vi "ListMenuActivation.vi"(0 "ListBox in":refnum<vi>, 1 "MenuRef":refnum<k9>, 2 "Point":T1) -> (14 "Menu Items":string[](array[string]), 19 "Discard Event?":bool)   [LabVIEW 2014, in "XListGraph.lvlib" / "XListGraph.xctl"]
uses:
  XListGraph.xctl
  <vilib>/Utility/miscctls.llb/LVPositionTypeDef.ctl
  <userlib>/_OpenG.lib/array/array.llb/Index 1D Array Elements (String)__ogtk.vi
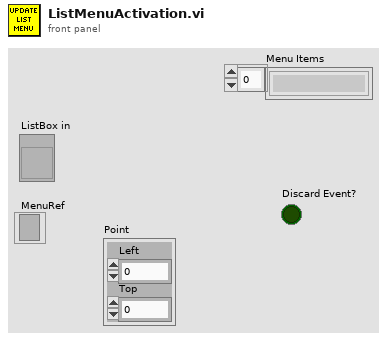
[diagram p1: front panel]
types:
  T1 = typedef "LVPositionTypeDef.ctl" = cluster{"Left":i32, "Top":i32}
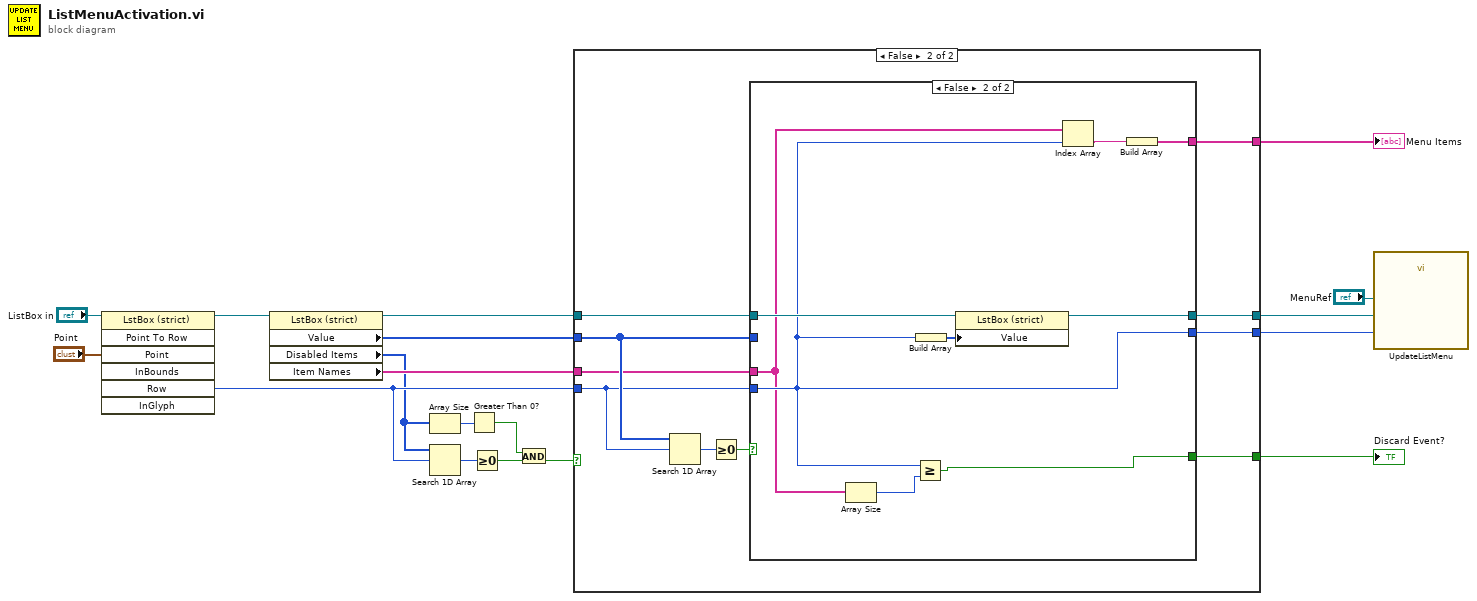
[diagram p0: block diagram]
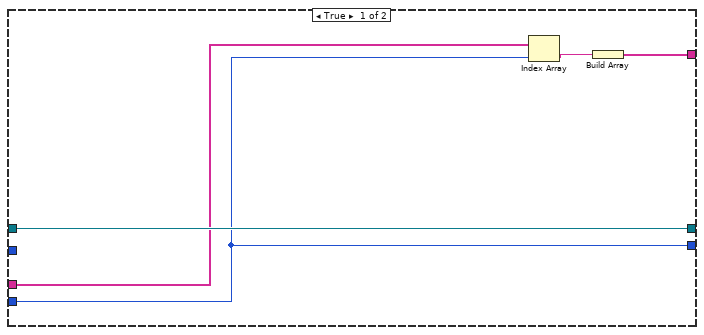
[diagram p2: hidden frame]
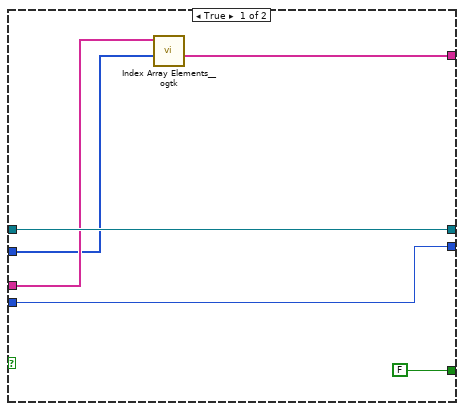
[diagram p3: hidden frame]
diagram:
  n1 = invoke on="Invoke Node" class="LstBox (strict)" method="Point To Row"(reference="ListBox in", "Point"="Point") -> (reference out=w15:refnum<vi>, "Row"=w11:i32)  [unwired: 5 in, 5 out]
  n2 = property class="LstBox (strict)"(reference=w15) -> (reference out=w14:refnum<vi>, "Value"=w18:i32[], "Disabled Items"=w4:i32[], "Item Names"=w16:string[])  [unwired: 1 in, 1 out]
  n3 = Array Size(array=w4) -> (size(s)=w2:i32)
  n4 = Search 1D Array(1D array=w4, element=w11) -> (index of element=w10:i32)  [unwired: 1 in]
  n5 = Greater Than 0?(x=w2) -> (x > 0?=w1:bool)
  n6 = Greater Or Equal To 0?(x=w10) -> (x >= 0?=w9:bool)
  n7 = And(x=w1, y=w9) -> (x .and. y?=w3:bool)
  n8 = case shown="False" w3 {
    tunnel: w18 -> [_ w31]
    tunnel: [w23 w33] -> w17
    tunnel: w16 -> [w21 w27]
    tunnel: w14 -> [w23 w32]
    tunnel: w11 -> [w20 w30]
    tunnel: [w20 w25] -> w7
    tunnel: [w19 w26] -> w6
    tunnel: [_ w24] -> w5
    frame True {
      n9 = Index Array(array=w21, index=w20) -> (element=w22:string)
      n10 = Build Array(w22) -> (w19:string[])
    }
    frame False {
      n11 = Search 1D Array(1D array=w31, element=w30) -> (index of element=w29:i32)  [unwired: 1 in]
      n12 = Greater Or Equal To 0?(x=w29) -> (x >= 0?=w28:bool)
      n13 = case shown="False" w28 {
        tunnel: [w39 w48] -> w33
        tunnel: w32 -> [w39 w47]
        tunnel: w31 -> [w37 _]
        tunnel: w30 -> [w35 w43]
        tunnel: w27 -> [w38 w42]
        tunnel: [w36 w44] -> w26
        tunnel: [w35 w43] -> w25
        tunnel: [FALSE w40] -> w24
        frame True {
          n14 = call-poly <userlib>:"Index Array Elements__ogtk.vi"("indices"=w37, "array"=w38) -> ("elements"=w36:string[])  [unwired: 9 in]
        }
        frame False {
          n15 = Array Size(array=w42) -> (size(s)=w41:i32)
          n16 = Greater Or Equal?(x=w43, y=w41) -> (x >= y?=w40:bool)
          n17 = Build Array(w43) -> (w46:i32[])
          n18 = property class="LstBox (strict)"(reference=w47, "Value"=w46) -> (reference out=w48:refnum<vi>)  [unwired: 1 in, 1 out]
          n19 = Index Array(array=w42, index=w43) -> (element=w45:string)
          n20 = Build Array(w45) -> (w44:string[])
        }
      }
    }
  }
  "Menu Items" <- w6
  "Discard Event?" <- w5
  n21 = call "UpdateListMenu.vi"("ListBox in"=w17, "MenuRef"="MenuRef", "PointedRow"=w7) -> ()  [unwired: 17 in]
